vi "NT_Array_Names_2020_Build_Season.vi"(10 "Name/Value":string, 11 "Subsystem":T1(ring)) -> (3 "Values":string)   [LabVIEW 2019]
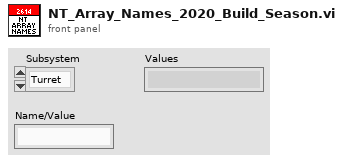
[diagram p1: front panel]
types:
  T1 = enum16{"Turret", "Magazine", "Intake", "Flywheel", "Drive", "Climb"}
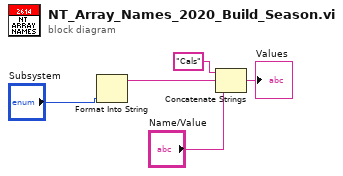
[diagram p0: block diagram]
diagram:
  n1 = Format Into String("Subsystem") -> (resulting string=w1:string)  [unwired: 3 in, 1 out]
  n2 = Concatenate Strings("Cals" ("string"), w1, "Name/Value") -> (→"Values":string)
